vi "Quadrature_Input_Example_Application.vi"() -> ()   [LabVIEW 2020]
panel:
  in  "error in (no error)":errorcluster
  in  "Phase Pairs":T1(ring)=enum."T7/T4: DIO6 + DIO7"
  in  "Device Type":string="LJM_dtANY"
  in  "Connection Type":string="LJM_ctANY"
  in  "Identifier":string="LJM_idANY"
  out "DeviceType Out":i32=7
  out "ConnectionType Out":i32=1
  out "error out":errorcluster
  out "Error String":string="No Error"
  in  "Encoder counts per revolution":i32=400
  out "Guage":dbl(knob) min=0.0 max=360.0 step=15.0 scale=0.0..360.0
  out "Degrees From Zero":i32
  out "Enc 2's Comp":dbl
  out "Enc Signed Int":dbl
  out "Revolutions":i32
  out "Direction":string="CC"
  out "Device Status":string="CLOSED"
  out "Open?":bool
  in  "stop":bool
  in  "Reset?":bool
  in  "Configure":bool
  # "T4 Capable DIO: DIO4, DIO5, DIO6, DIO7, DIO8, DIO9 (aka FIO4, FIO5, FIO6, FIO7, EIO0, EIO1)\n \nT7 Capable DIO: DIO0, DIO1, DIO2, DIO3, DIO6, DIO7 (aka FIO0, FIO1, FIO2, FIO3, FIO6, FIO7)\n\nThe channels must be used in one of the consecutive pairs that can be selected below in \"Phase Pairs\" .The even channel is Phase A and odd channel is Phase B of the encoder.\n\nMake sure to set how many counts per revolution for the encoder and the necessary device credentials, then click Configure/Start to begin.\n\nThe device can be reconfigured at anytime with the Configure/Start button"
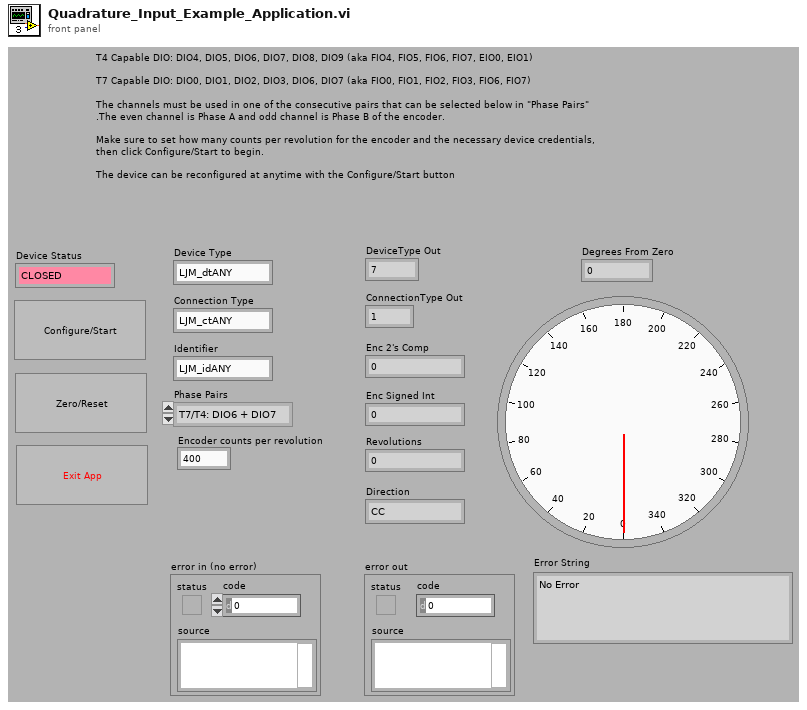
[diagram p1: front panel]
types:
  T1 = enum16{"T7: DIO0 + DIO1", "T7: DIO2 + DIO3", "T7/T4: DIO6 + DIO7", "T4: DIO4 + DIO5", "T4: DIO8 + DIO9"}
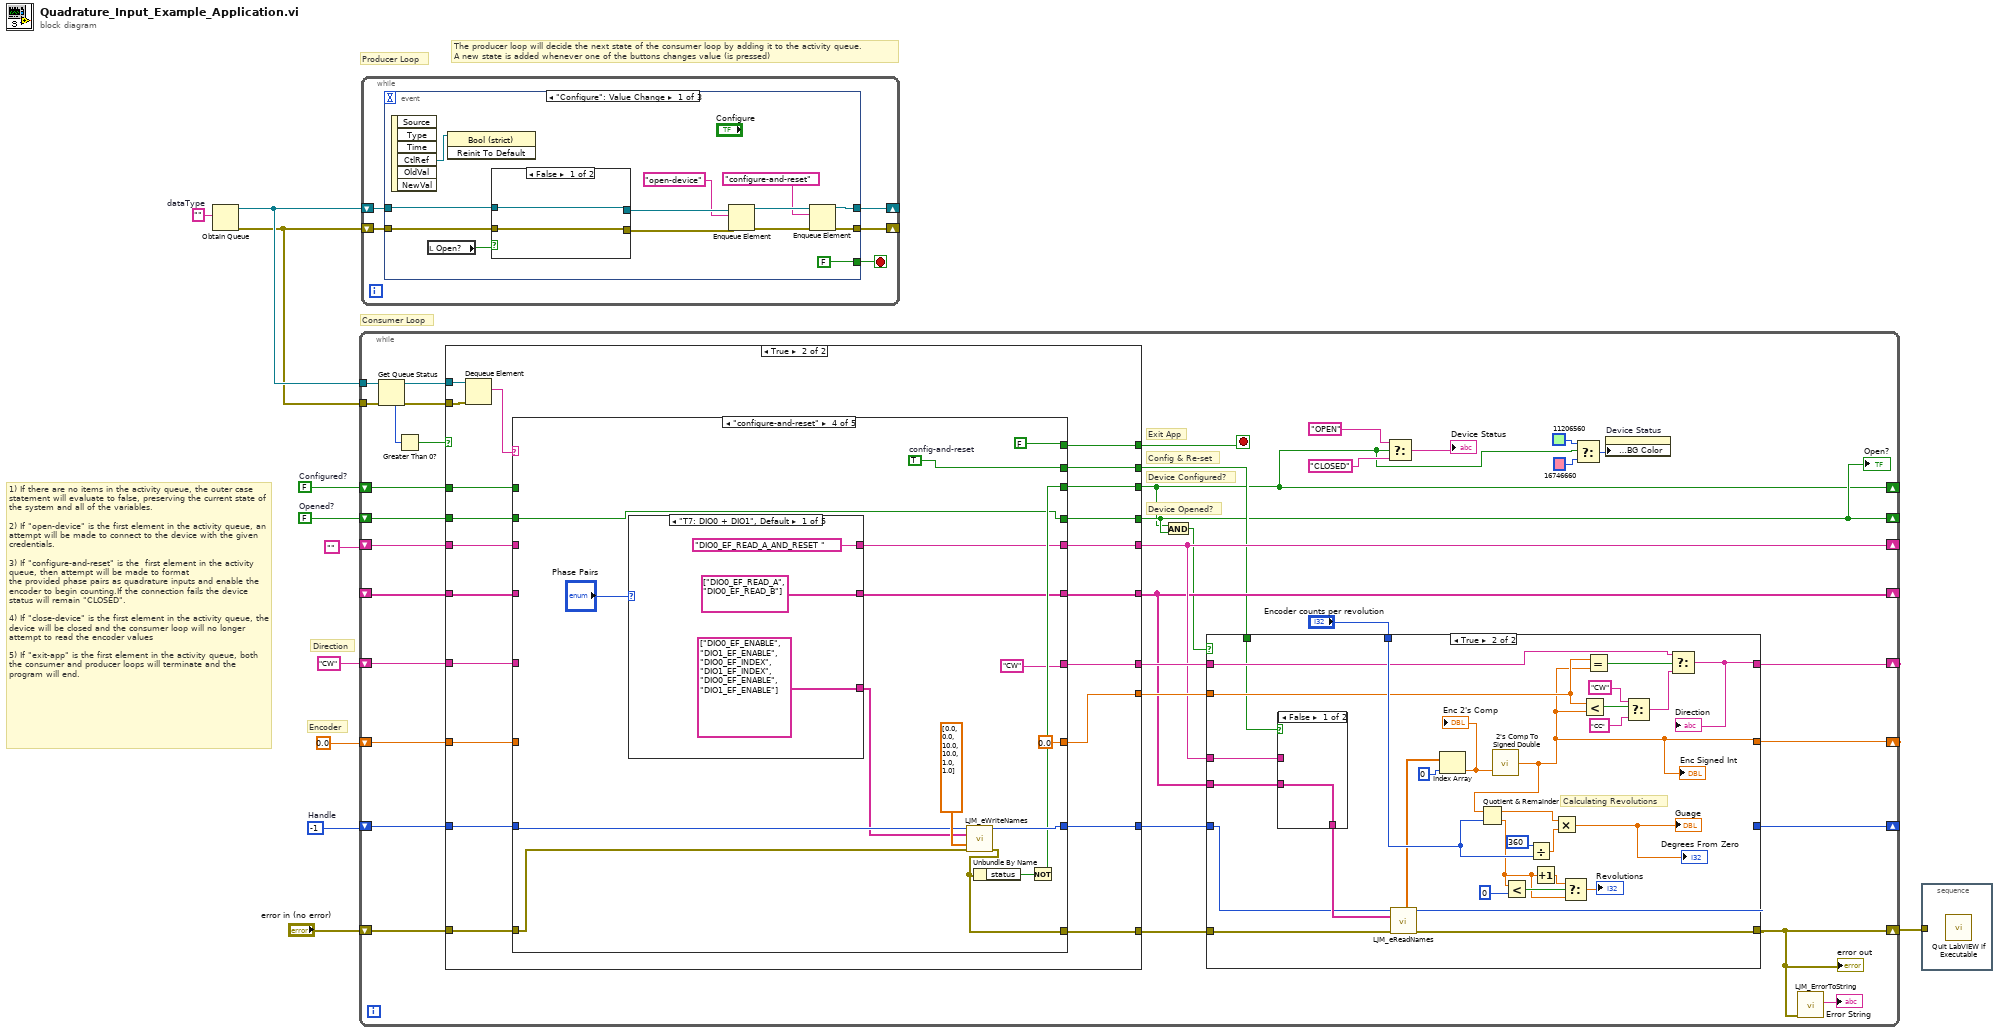
[diagram p0: block diagram]
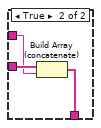
[diagram p3: hidden frame]
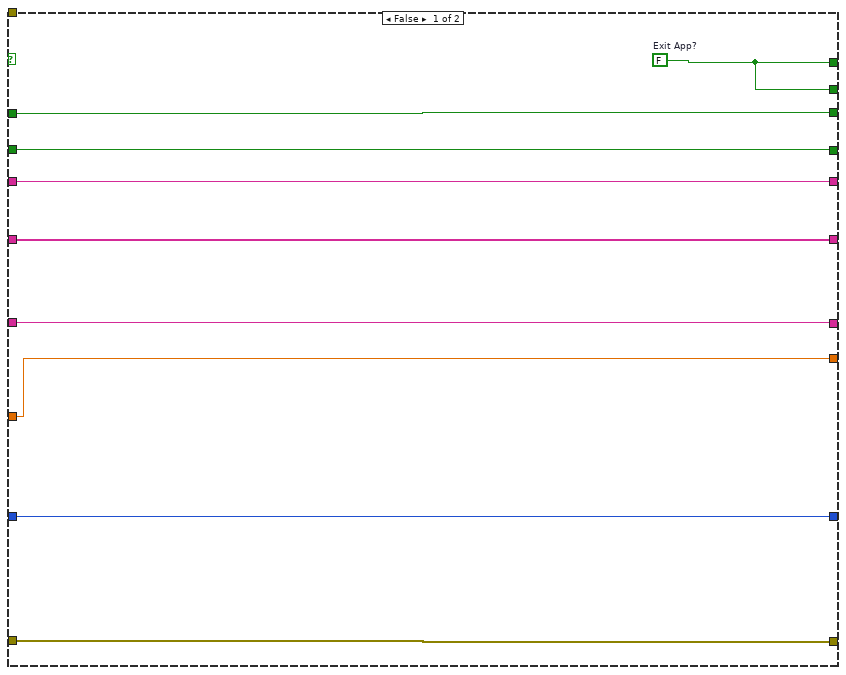
[diagram p4: hidden frame]
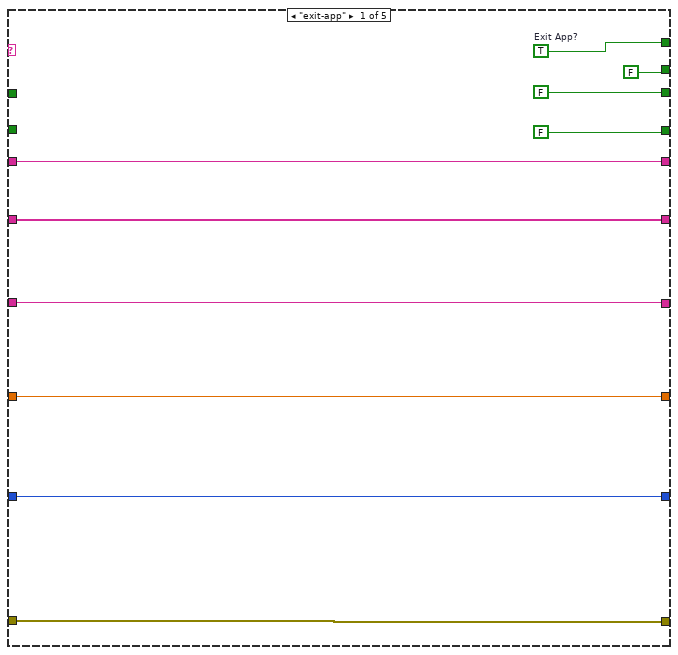
[diagram p5: hidden frame]
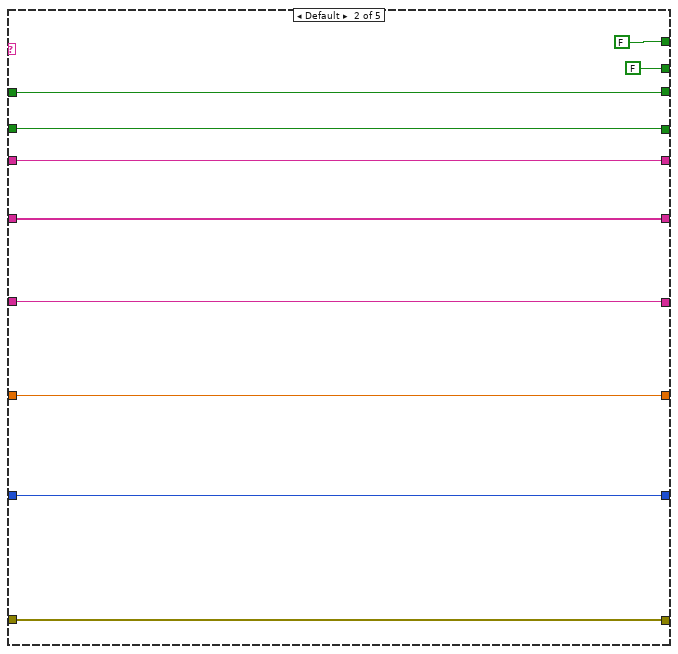
[diagram p6: hidden frame]
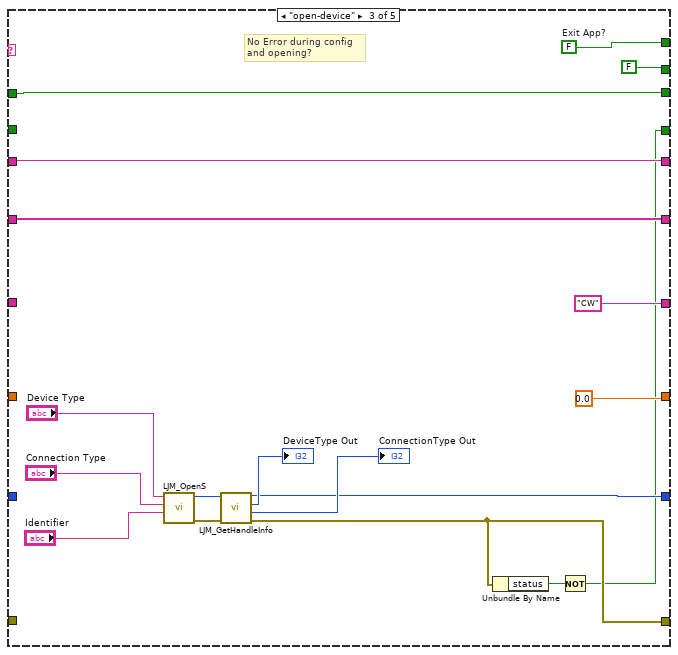
[diagram p7: hidden frame]
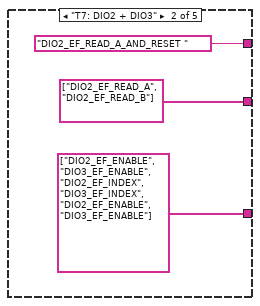
[diagram p8: hidden frame]
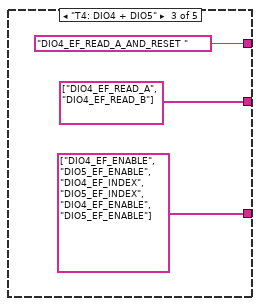
[diagram p9: hidden frame]
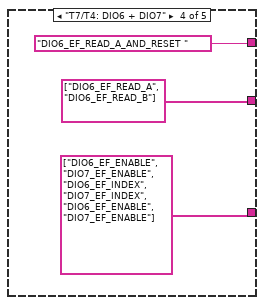
[diagram p10: hidden frame]
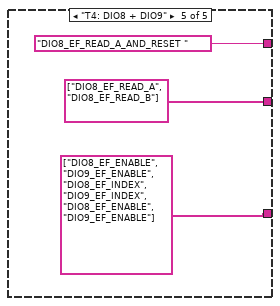
[diagram p11: hidden frame]
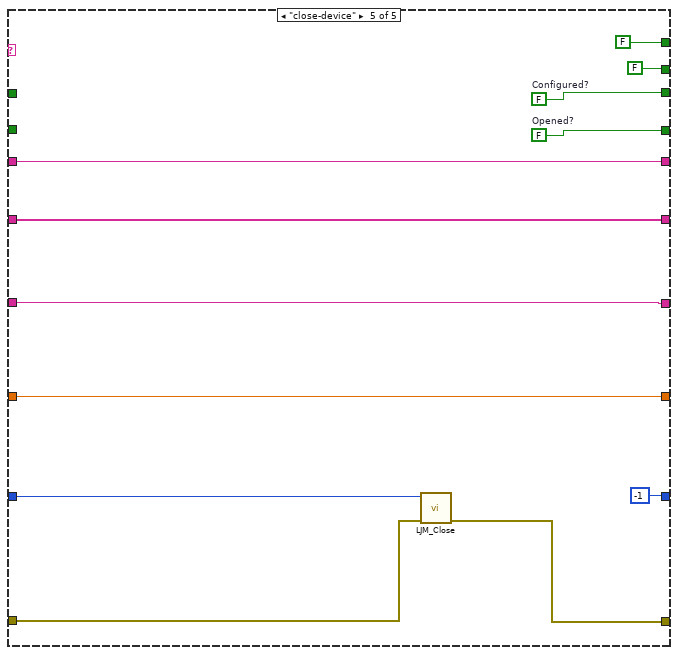
[diagram p12: hidden frame]
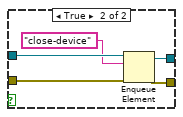
[diagram p13: hidden frame]
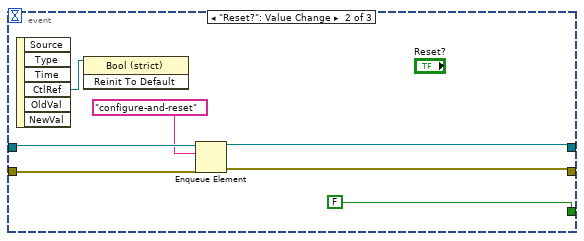
[diagram p14: hidden frame]
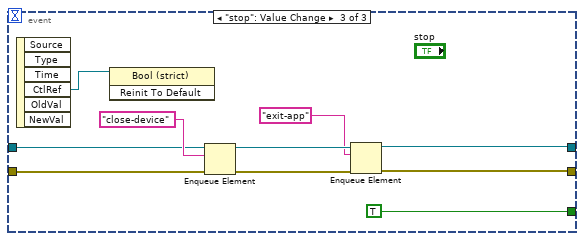
[diagram p15: hidden frame]
diagram:
  w2 = -1  # Handle
  w3 = FALSE  # Opened?
  w9 = FALSE  # Configured?
  w11 = ""  # dataType
  # "1) If there are no items in the activity queue, the outer case statement will evaluate to false, preserving the current state of the system and all of the variables.     \n\n2) If \"open-device\" is the first element in the activity queue, an attempt will be made to connect to the device with the given credentials. \n\n3) If \"configure-and-reset\" is the  first element in the activity queue, then attempt will be made to format\nthe provided phase pairs as quadrature inputs and enable the encoder to begin counting.If the connection fails the device status will remain \"CLOSED\".\n\n4) If \"close-device\" is the first element in the activity queue, the device will be closed and the consumer loop will no longer attempt to read the encoder values\n\n5) If \"exit-app\" is the first element in the activity queue, both the consumer and producer loops will terminate and the program will end."
  # "The producer loop will decide the next state of the consumer loop by adding it to the activity queue. \nA new state is added whenever one of the buttons changes value (is pressed)"
  # "Encoder"
  # "Direction"
  # "Consumer Loop"
  # "Producer Loop"
  n1 = Obtain Queue(element data type=w11) -> (queue out=w5:refnum<queue>, error out=w4:errorcluster)  [unwired: 4 in, 1 out]
  n2 = while {
    tunnel: w5 -> [w48]
    tunnel: w4 -> [w47]
    shift-right: [w34] -> w1
    shift-left: "error in (no error)" -> [w42]
    shift-right: [w31] -> _
    shift-left: w2 -> [w40]
    shift-right: [w25] -> _
    shift-left: "" -> [w26]
    shift-right: [w24] -> _
    shift-left: _ -> [w41]
    shift-right: [w12] -> _
    shift-left: w9 -> [w38]
    shift-right: [w33] -> _
    shift-left: "CW" -> [w32]
    shift-right: [w30] -> _
    shift-left: 0.0 -> [w28]
    shift-right: [w13] -> _
    shift-left: w3 -> [w19]
    stop <- w23 stop-if-true
    # "Device Opened?"
    # "Device Configured?"
    # "Config & Re-set"
    # "Exit App"
    n3 = Get Queue Status(queue=w48, error in (no error)=w47) -> (queue out=w46:refnum<queue>, error out=w45:errorcluster, # elements in queue=w43:i32)  [unwired: 1 in, 5 out]
    n4 = Greater Than 0?(x=w43) -> (x > 0?=w44:bool)
    n5 = case shown="True" w44 {
      tunnel: w46 -> [_ w116]
      tunnel: w45 -> [_ w115]
      tunnel: [w87 w108] -> w23
      tunnel: w42 -> [w93 w113]
      tunnel: [w93 w112] -> w36
      tunnel: [w94 w111] -> w35
      tunnel: [w95 w110] -> w25
      tunnel: [w89 w109] -> w24
      tunnel: w26 -> [w95 w106]
      tunnel: w41 -> [w89 w105]
      tunnel: w40 -> [w94 w107]
      tunnel: w38 -> [w92 w104]
      tunnel: [w92 w103] -> w12
      tunnel: w32 -> [w91 w102]
      tunnel: [w91 w101] -> w29
      tunnel: w28 -> [w90 w100]
      tunnel: [w90 w99] -> w27
      tunnel: w19 -> [w88 w98]
      tunnel: [w88 w97] -> w13
      tunnel: [w87 w96] -> w17
      frame False {
        w87 = FALSE  # Exit App?
      }
      frame True {
        n6 = Dequeue Element(queue=w116, error in (no error)=w115) -> (element=w114:string)  [unwired: 1 in, 3 out]
        n7 = case shown="\"configure-and-reset\"" w114 {
          tunnel: [w126 FALSE w147 FALSE FALSE] -> w108
          tunnel: w113 -> [w122 w129 _ w166 w197]
          tunnel: [w122 w129 w141 w157 w193] -> w112
          tunnel: [w123 w130 w140 w165 -1] -> w111
          tunnel: [w125 w134 w142 w160 w195] -> w110
          tunnel: [w124 w133 w143 w155 w194] -> w109
          tunnel: w107 -> [w123 w130 _ w167 w196]
          tunnel: w106 -> [w125 w134 w142 _ w195]
          tunnel: w105 -> [w124 w133 w143 _ w194]
          tunnel: w104 -> [_ w136 w138 _ _]
          tunnel: [FALSE ("Exit App?") w136 w138 w164 w189] -> w103
          tunnel: [w120 w132 "CW" "CW" w192] -> w101
          tunnel: w102 -> [w120 w132 _ _ w192]
          tunnel: [w119 w131 0.0 0.0 w191] -> w99
          tunnel: w100 -> [w119 w131 _ _ w191]
          tunnel: w98 -> [_ w135 _ w159 _]
          tunnel: [FALSE ("Exit App?") w135 w139 w159 w188] -> w97
          tunnel: [FALSE ("Exit App?") FALSE ("Exit App?") FALSE ("Exit App?") w156 FALSE ("Exit App?")] -> w96
          frame "exit-app" {
            w126 = TRUE  # Exit App?
          }
          frame Default {
          }
          frame "open-device" {
            w147 = FALSE  # Exit App?
            # "No Error during config\nand opening?"
            n8 = call "LJM_OpenS.vi"("Identifier"="Identifier", "ConnectionType"="Connection Type", "DeviceType"="Device Type") -> ("error out"=w148:errorcluster, "Handle"=w149:i32)  [unwired: 7 in]
            n9 = call "LJM_GetHandleInfo.vi"("error in"=w148, "Handle In"=w149) -> ("error out"=w141:errorcluster, "ConnectionType"=→"ConnectionType Out":i32, "DeviceType"=→"DeviceType Out":i32, "Handle Out"=w140:i32)  [unwired: 2 in, 4 out]
            n10 = Unbundle By Name(w141) -> ("status"=w146:bool)
            n11 = Not(x=w146) -> (.not. x?=w139:bool)
          }
          frame "configure-and-reset" {
            w156 = TRUE  # config-and-reset
            n12 = case shown="\"T7: DIO0 + DIO1\", Default" "Phase Pairs" {
              tunnel: [string[] ["DIO0_EF_READ_A", "DIO0_EF_READ_B"] string[] ["DIO2_EF_READ_A", "DIO2_EF_READ_B"] string[] ["DIO4_EF_READ_A", "DIO4_EF_READ_B"] string[] ["DIO6_EF_READ_A", "DIO6_EF_READ_B"] string[] ["DIO8_EF_READ_A", "DIO8_EF_READ_B"]] -> w155
              tunnel: [string[] ["DIO0_EF_ENABLE", "DIO1_EF_ENABLE", "DIO0_EF_INDEX", "DIO1_EF_INDEX", "DIO0_EF_ENABLE", "DIO1_EF_ENABLE"] string[] ["DIO2_EF_ENABLE", "DIO3_EF_ENABLE", "DIO2_EF_INDEX", "DIO3_EF_INDEX", "DIO2_EF_ENABLE", "DIO3_EF_ENABLE"] string[] ["DIO4_EF_ENABLE", "DIO5_EF_ENABLE", "DIO4_EF_INDEX", "DIO5_EF_INDEX", "DIO4_EF_ENABLE", "DIO5_EF_ENABLE"] string[] ["DIO6_EF_ENABLE", "DIO7_EF_ENABLE", "DIO6_EF_INDEX", "DIO7_EF_INDEX", "DIO6_EF_ENABLE", "DIO7_EF_ENABLE"] string[] ["DIO8_EF_ENABLE", "DIO9_EF_ENABLE", "DIO8_EF_INDEX", "DIO9_EF_INDEX", "DIO8_EF_ENABLE", "DIO9_EF_ENABLE"]] -> w163
              tunnel: ["DIO0_EF_READ_A_AND_RESET " "DIO2_EF_READ_A_AND_RESET " "DIO4_EF_READ_A_AND_RESET " "DIO6_EF_READ_A_AND_RESET " "DIO8_EF_READ_A_AND_RESET "] -> w160
              frame "T7: DIO0 + DIO1", Default {
              }
              frame "T7: DIO2 + DIO3" {
              }
              frame "T4: DIO4 + DIO5" {
              }
              frame "T7/T4: DIO6 + DIO7" {
              }
              frame "T4: DIO8 + DIO9" {
              }
            }
            n13 = call "LJM_eWriteNames.vi"("Handle In"=w167, "aNames"=w163, "aValuesIn"=dbl[] [0.0, 0.0, 10.0, 10.0, 1.0, 1.0], "error in"=w166) -> ("Handle Out"=w165:i32, "error out"=w157:errorcluster)  [unwired: 9 in, 1 out]
            n14 = Unbundle By Name(w157) -> ("status"=w168:bool)
            n15 = Not(x=w168) -> (.not. x?=w164:bool)
          }
          frame "close-device" {
            w188 = FALSE  # Opened?
            w189 = FALSE  # Configured?
            n16 = call "LJM_Close.vi"("error in"=w197, "Handle"=w196) -> ("error out"=w193:errorcluster)  [unwired: 9 in]
          }
        }
      }
    }
    "Open?" <- w13
    n17 = And(x=w12, y=w13) -> (x .and. y?=w18:bool)
    n18 = case shown="True" w18 {
      tunnel: "Encoder counts per revolution" -> [_ w82]
      tunnel: w36 -> [w51 w70]
      tunnel: w35 -> [w52 w65]
      tunnel: [w51 w69] -> w34
      tunnel: w24 -> [_ w68]
      tunnel: w25 -> [_ w67]
      tunnel: [w49 w66] -> w33
      tunnel: [w52 w60] -> w31
      tunnel: [w50 w53] -> w30
      tunnel: w29 -> [w49 w64]
      tunnel: w27 -> [w50 w63]
      tunnel: w17 -> [_ w62]
      frame False {
      }
      frame True {
        # "Calculating Revolutions"
        n19 = case shown="False" w62 {
          tunnel: w67 -> [_ w85]
          tunnel: w68 -> [w83 w86]
          tunnel: [w83 w84] -> w77
          frame False {
          }
          frame True {
            n20 = Build Array (concatenate)(w86, w85) -> (w84:string[])
          }
        }
        n21 = call "LJM_eReadNames.vi"("Handle In"=w65, "aNames"=w77, "error in"=w70) -> ("Handle Out"=w60:i32, "aValuesOut"=w79:dbl[], "error out"=w69:errorcluster)  [unwired: 9 in, 1 out]
        n22 = Index Array(array=w79, index=0) -> (element=w54:dbl)
        "Enc 2's Comp" <- w54
        n23 = call "2's Comp To Signed Double.vi"("2's ccomp"=w54) -> ("Signed Double"=w53:dbl)  [unwired: 1 in]
        "Enc Signed Int" <- w53
        n24 = Quotient & Remainder(x=w53, y=w82) -> (x-y*floor(x/y)=w61:dbl, floor(x/y)=w55:dbl)
        n25 = Less?(x=w55, y=0) -> (x < y?=w59:bool)
        n26 = Divide(x=360, y=w82) -> (x/y=w80:dbl)
        n27 = Increment(x=w55) -> (x+1=w56:dbl)
        n28 = Multiply(x=w61, y=w80) -> (x*y=→"Guage" →"Degrees From Zero":dbl)
        n29 = Select(t=w56, s=w59, f=w55) -> (s? t:f=→"Revolutions":dbl)
        n30 = Less?(x=w63, y=w53) -> (x < y?=w75:bool)
        n31 = Equal?(x=w63, y=w53) -> (x = y?=w73:bool)
        n32 = Select(t="CW", s=w75, f="CC") -> (s? t:f=w72:string)
        n33 = Select(t=w64, s=w73, f=w72) -> (s? t:f=w66:string)
        "Direction" <- w66
      }
    }
    "error out" <- w34
    n34 = Select(t="OPEN", s=w12, f="CLOSED") -> (s? t:f=→"Device Status":string)
    n35 = Select(t=u32 11206560, s=w12, f=u32 16746660) -> (s? t:f=w16:u32)
    n36 = property on="Device Status" class="Str"("Text.Text Colors:BG Color"=w16) -> ()  [unwired: 2 in, 2 out]
    n37 = call "LJM_ErrorToString.vi"("error in"=w34) -> ("String"=→"Error String":string)  [unwired: 10 in]
  }
  n38 = while {
    shift-right: [w199] -> _
    shift-left: w5 -> [w202]
    shift-right: [w198] -> _
    shift-left: w4 -> [w201]
    stop <- w200 stop-if-true
    n39 = event shown="[0] \"Configure\": Value Change" {
      selector: _ -> [_ _ _]
      dyn-events: _ -> [_ _ _]
      timeout: _ -> [_ _ _]
      tunnel: w202 -> [w214 w228 w238]
      tunnel: w201 -> [w215 w229 w237]
      tunnel: [FALSE FALSE TRUE] -> w200
      tunnel: [w206 w224 w233] -> w199
      tunnel: [w205 w223 w234] -> w198
      event "Configure": Value Change {
        n40 = event-data() -> ("CtlRef"=w209:refnum<vi>)  [unwired: 1 in, 5 out]
        n41 = local read "Open?"() -> (w203:bool)
        n42 = invoke class="Bool (strict)" method="Reinit To Default"(reference=w209) -> ()  [unwired: 2 in, 3 out]
        n43 = case shown="False" w203 {
          tunnel: w215 -> [w216 w222]
          tunnel: w214 -> [w217 w221]
          tunnel: [w217 w219] -> w213
          tunnel: [w216 w218] -> w212
          frame False {
          }
          frame True {
            n44 = Enqueue Element(queue=w221, element="close-device", error in (no error)=w222) -> (queue out=w219:refnum<queue>, error out=w218:errorcluster)  [unwired: 1 in, 1 out]
          }
        }
        n45 = Enqueue Element(queue=w213, element="open-device", error in (no error)=w212) -> (queue out=w208:refnum<queue>, error out=w207:errorcluster)  [unwired: 1 in, 1 out]
        n46 = Enqueue Element(queue=w208, element="configure-and-reset", error in (no error)=w207) -> (queue out=w206:refnum<queue>, error out=w205:errorcluster)  [unwired: 1 in, 1 out]
      }
      event "Reset?": Value Change {
        n47 = event-data() -> ("CtlRef"=w225:refnum<vi>)  [unwired: 1 in, 5 out]
        n48 = invoke class="Bool (strict)" method="Reinit To Default"(reference=w225) -> ()  [unwired: 2 in, 3 out]
        n49 = Enqueue Element(queue=w228, element="configure-and-reset", error in (no error)=w229) -> (queue out=w224:refnum<queue>, error out=w223:errorcluster)  [unwired: 1 in, 1 out]
      }
      event "stop": Value Change {
        n50 = event-data() -> ("CtlRef"=w230:refnum<vi>)  [unwired: 1 in, 5 out]
        n51 = invoke class="Bool (strict)" method="Reinit To Default"(reference=w230) -> ()  [unwired: 2 in, 3 out]
        n52 = Enqueue Element(queue=w238, element="close-device", error in (no error)=w237) -> (queue out=w236:refnum<queue>, error out=w235:errorcluster)  [unwired: 1 in, 1 out]
        n53 = Enqueue Element(queue=w236, element="exit-app", error in (no error)=w235) -> (queue out=w233:refnum<queue>, error out=w234:errorcluster)  [unwired: 1 in, 1 out]
      }
    }
  }
  n54 = stacked-sequence {
    tunnel: w1 -> [_]
    frame #0 {
      n55 = call "Quit LabVIEW if Executable.vi"() -> ()  [unwired: 1 in]
    }
  }
